vi "LoadConfigPhospho.vi"(8 "configuration file path":path caption="chemin du fichier de configuration") -> (0 "Acquisition properties":T2, 1 "Associated files":T1, 3 "Pulse properties":T3={"N pulses"=0, "Samples"=0, "Last samples"=0, "AO pulse ticks"=0, "Skip samples"=0, "N samples/decay"=0, "Sliding Step \n(nb pulses)"=0, "Slidiing window\n (nb pulses)"=0, "Interpoints \ninterval (ms)"=100.0, "Mean and Time-Lapsed on Point Number"=0, "Number of points"=0, "Repeat \neach point"=8, "Oxygen dye type"=10106, "Interpulse Interval"=0.0, "N samples/ decay min"=0} {"Oxygen dye type" items=["PtP-C343 (30 kDa)", "PtP-C343 (65 KDa)"]; "Repeat \neach point" min=2 step=1})   [LabVIEW 2013, in "Phosphorescence - Mode.lvlib"]
uses:
  Phosphorescence - Mode.lvlib
  <vilib>/Utility/config.llb/Read Key (I32).vi
  <vilib>/Utility/config.llb/Read Key (Double).vi
  <vilib>/Utility/config.llb/Read Key (String).vi
  <vilib>/Utility/config.llb/NI_LVConfig.lvlib
  File management.lvlib
panel:
  out "Wait":i32=30
  in  "TDMS path":string
  out "N samples/ decay min":i32
  out "Interpulse Interval":dbl
  in  "Oxygen dye type":i16(ring)=10106 items=["PtP-C343 (30 kDa)", "PtP-C343 (65 KDa)"]
  in  "Timing file":string
  in  "Results file":string
  in  "Raw Images file":string[][](array[string])
  in  "Repeat \neach point":i32
  in  "Number of points":i32
  in  "Mean and Time-Lapsed on Point Number":i32
  in  "Interpoints \ninterval (ms)":dbl
  in  "Reference text file":string
  in  "Reference image files":string[](array[string])
  in  "Mean and fit file":string
  out "Selection coordinates":dbl[](array[numeric])=[0.5875, 0.6937500000000001, 0.9437500000000001, 0.9750000000000001, 0.5875, 0.7364583333333334, 0.5916666666666667, 0.696875, 0.9333333333333333, 0.6937500000000001, 0.9437500000000001, 0.7208333333333333, 0.7822916666666666, 0.9750000000000001, 0.7562500000000001, 0.971875, 0.5875, 0.7364583333333334]
  out "Pictures coordinates":dbl[](array[numeric])=[0.5875, 0.6937500000000001, 0.9437500000000001, 0.9750000000000001, 0.5875, 0.7364583333333334, 0.5916666666666667, 0.696875, 0.9333333333333333, 0.6937500000000001, 0.9437500000000001, 0.7208333333333333, 0.7822916666666666, 0.9750000000000001, 0.7562500000000001, 0.971875, 0.5875, 0.7364583333333334]
  out "pwr_rel":dbl(slide)=0.01 min=0.01 max=1.0 step=0.005 scale=0.01..1.0 scale format="%.2f"
  out "Channel Acquired":i32 min=0 max=1 step=1
  out "scan rate (kHz)":dbl=1000.0 caption="Rate (kHz)"
  out "Last samples":i32=5
  out "Sliding Step \n(nb pulses)":i32=8 min=2 step=1
  out "Slidiing window\n (nb pulses)":i32=8 min=2 step=1
  out "Skip samples":i32=12
  out "Samples":i32=1500 caption="Total scans"
  out "N samples/decay":i32=150
  out "pulse ticks":i32=8 min=2 step=1
  out "N pulses":i32=10
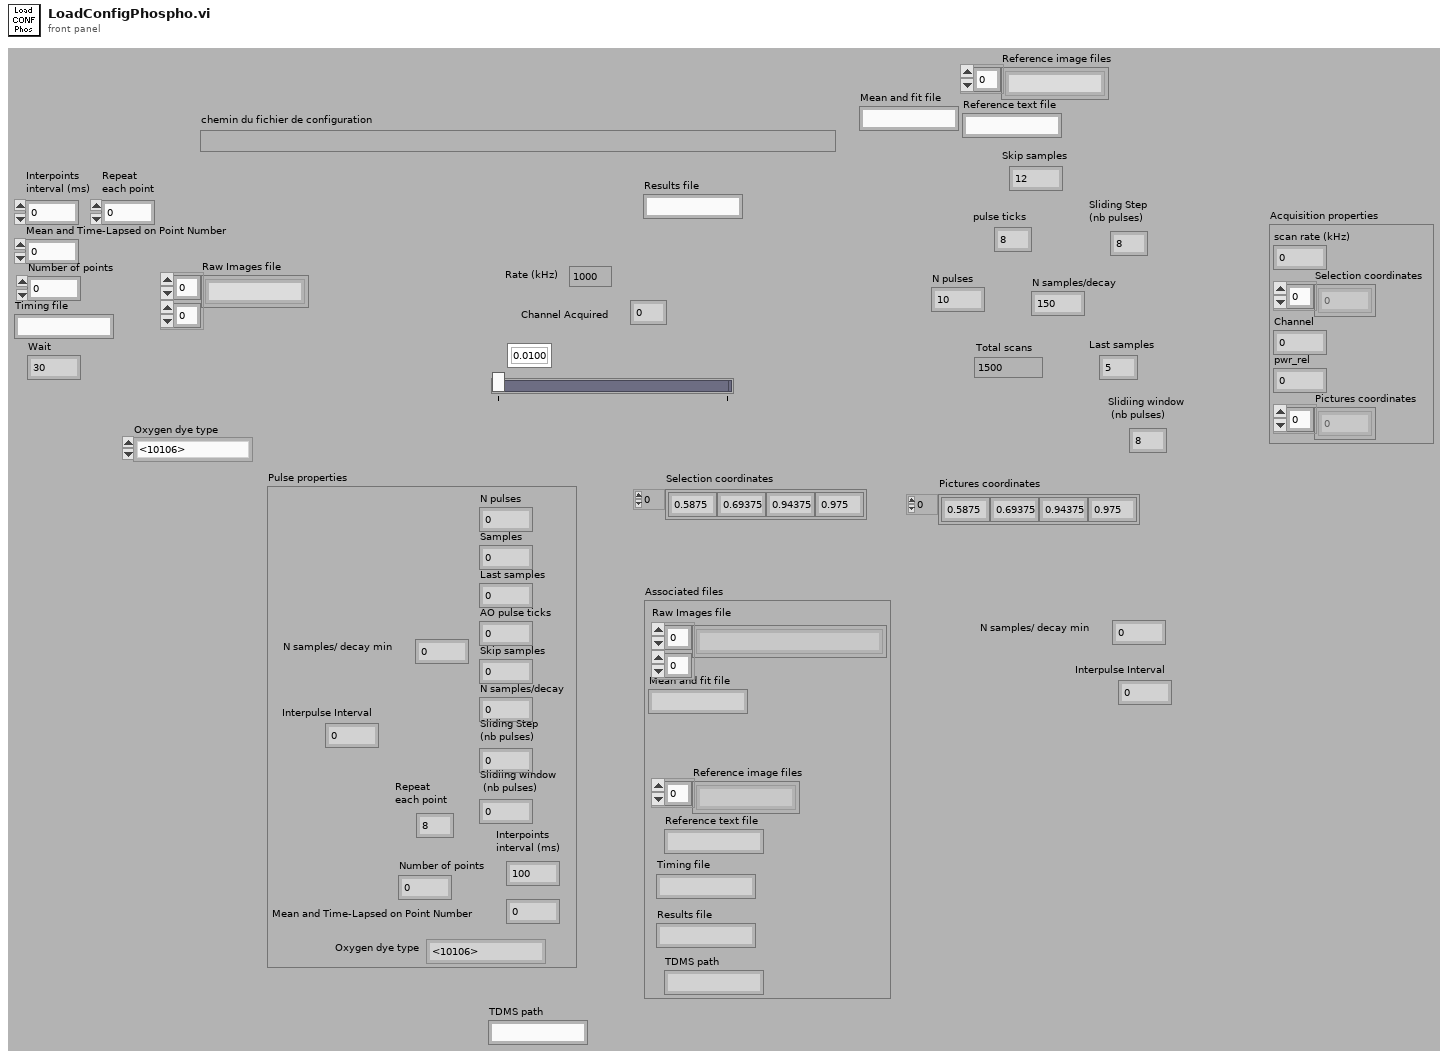
[diagram p1: front panel]
types:
  T1 = cluster{"Mean and fit file":string, "Reference image files":string[], "Reference text file":string, "Results file":string, "Timing file":string, "Raw Images file":string[][], "TDMS path":string}
  T2 = cluster{"scan rate (kHz)":dbl, "Selection coordinates":dbl[], "Channel":i32, "pwr_rel":dbl, "Pictures coordinates":dbl[]}
  T3 = cluster{"N pulses":i32, "Samples":i32, "Last samples":i32, "AO pulse ticks":i32, "Skip samples":i32, "N samples/decay":i32, "Sliding Step \n(nb pulses)":i32, "Slidiing window\n (nb pulses)":i32, "Interpoints \ninterval (ms)":dbl, "Mean and Time-Lapsed on Point Number":i32, "Number of points":i32, "Repeat \neach point":i32, "Oxygen dye type":i16, "Interpulse Interval":dbl, "N samples/ decay min":i32}
  T4 = typedef "NI_LVConfig.lvlib/Config Data RefNum.ctl" = refnum<k1>
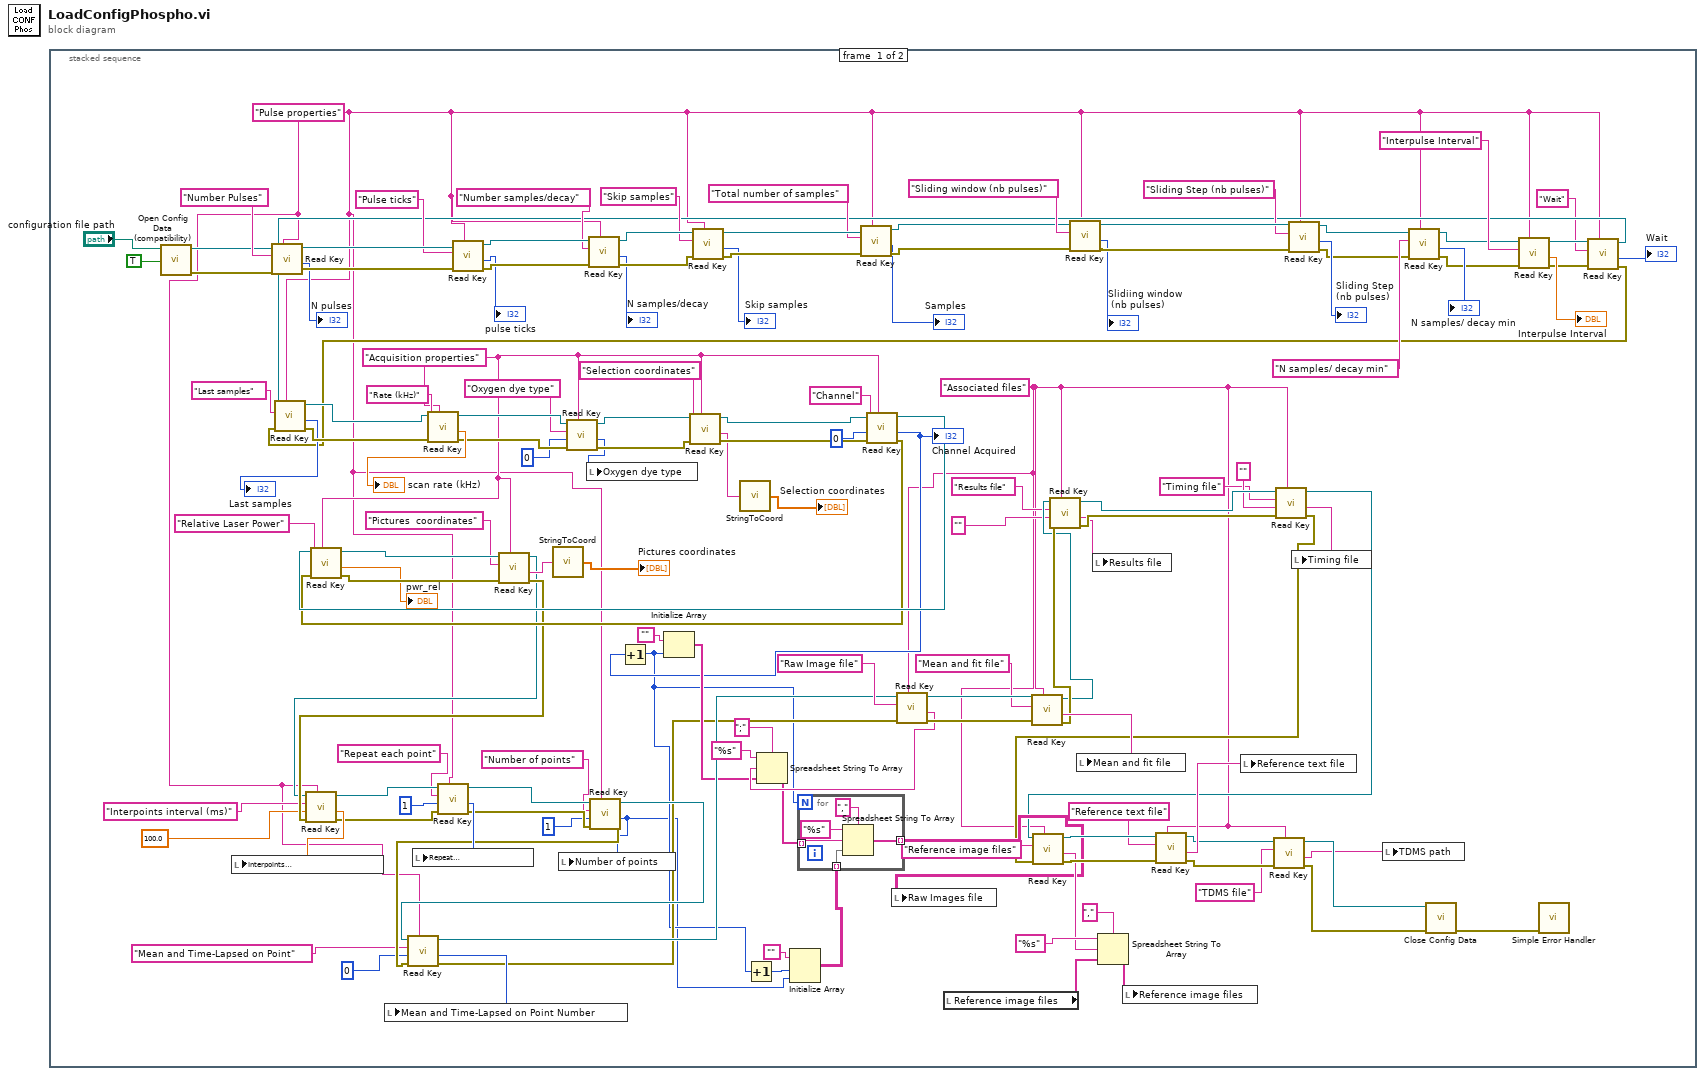
[diagram p0: block diagram]
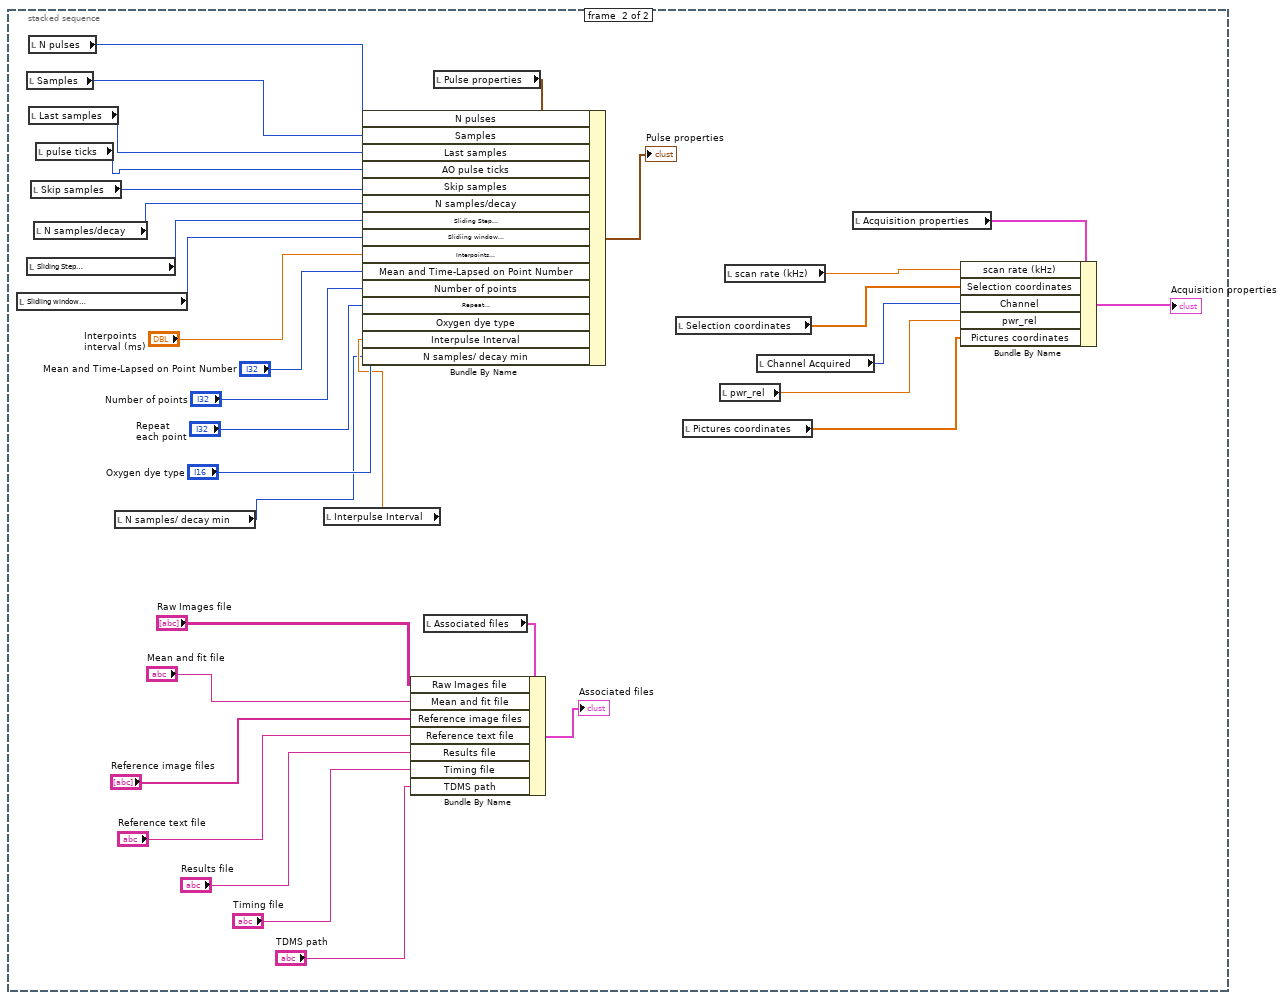
[diagram p2: hidden frame]
diagram:
  n1 = stacked-sequence {
    frame #0 {
      w9 = "Associated files" ("key")
      w29 = "Acquisition properties" ("section")
      w1 = "Pulse properties" ("section")
      n2 = call <vilib>:"Open Config Data (compatibility).vi"("create file if necessary (T)"=TRUE ("create file if necessary? (T)"), "configuration file path"="configuration file path") -> ("error out"=w113:errorcluster, "refnum"=w112:T4)  [unwired: 7 in, 1 out]
      n3 = call-poly <vilib>:"Read Key.vi"("section"=w1, "error in (no error)"=w113, "key"="Number Pulses", "refnum"=w112) -> ("error out"=w124:errorcluster, "value"=→"N pulses":i32, "refnum out"=w119:T4)  [unwired: 1 in, 4 out]
      n4 = call-poly <vilib>:"Read Key.vi"("section"=w1, "error in (no error)"=w124, "key"="Pulse ticks", "refnum"=w119) -> ("error out"=w123:errorcluster, "value"=→"pulse ticks":i32, "refnum out"=w118:T4)  [unwired: 1 in, 4 out]
      n5 = call-poly <vilib>:"Read Key.vi"("section"=w1, "error in (no error)"=w123, "key"="Number samples/decay", "refnum"=w118) -> ("error out"=w122:errorcluster, "value"=→"N samples/decay":i32, "refnum out"=w121:T4)  [unwired: 1 in, 4 out]
      n6 = call-poly <vilib>:"Read Key.vi"("section"=w1, "error in (no error)"=w122, "key"="Skip samples", "refnum"=w121) -> ("error out"=w130:errorcluster, "value"=→"Skip samples":i32, "refnum out"=w129:T4)  [unwired: 1 in, 4 out]
      n7 = call-poly <vilib>:"Read Key.vi"("section"=w1, "error in (no error)"=w130, "key"="Total number of samples", "refnum"=w129) -> ("error out"=w107:errorcluster, "value"=→"Samples":i32, "refnum out"=w108:T4)  [unwired: 1 in, 4 out]
      n8 = local read "Reference image files"() -> (w85:string[])
      n9 = call-poly <vilib>:"Read Key.vi"("section"=w1, "error in (no error)"=w107, "key"="Sliding window (nb pulses)", "refnum"=w108) -> ("error out"=w142:errorcluster, "value"=→"Slidiing window\n (nb pulses)":i32, "refnum out"=w141:T4)  [unwired: 1 in, 4 out]
      n10 = call-poly <vilib>:"Read Key.vi"("section"=w1, "error in (no error)"=w142, "key"="Sliding Step (nb pulses)", "refnum"=w141) -> ("error out"=w18:errorcluster, "value"=→"Sliding Step \n(nb pulses)":i32, "refnum out"=w19:T4)  [unwired: 1 in, 4 out]
      n11 = call-poly <vilib>:"Read Key.vi"("section"=w1, "error in (no error)"=w18, "key"="N samples/ decay min", "refnum"=w19) -> ("error out"=w17:errorcluster, "value"=→"N samples/ decay min":i32, "refnum out"=w20:T4)  [unwired: 1 in, 4 out]
      n12 = call-poly <vilib>:"Read Key.vi"("section"=w1, "error in (no error)"=w17, "key"="Interpulse Interval", "refnum"=w20) -> ("error out"=w5:errorcluster, "value"=→"Interpulse Interval":dbl, "refnum out"=w3:T4)  [unwired: 1 in, 4 out]
      n13 = call-poly <vilib>:"Read Key.vi"("section"=w1, "error in (no error)"=w5, "key"="Wait", "refnum"=w3) -> ("error out"=w6:errorcluster, "value"=→"Wait":i32, "refnum out"=w4:T4)  [unwired: 2 in, 3 out]
      n14 = call-poly <vilib>:"Read Key.vi"("section"=w1, "error in (no error)"=w6, "key"="Last samples", "refnum"=w4) -> ("error out"=w144:errorcluster, "value"=→"Last samples":i32, "refnum out"=w126:T4)  [unwired: 1 in, 4 out]
      n15 = call-poly <vilib>:"Read Key.vi"("section"=w29, "error in (no error)"=w144, "key"="Rate (kHz)", "refnum"=w126) -> ("error out"=w33:errorcluster, "value"=→"scan rate (kHz)":dbl, "refnum out"=w30:T4)  [unwired: 2 in, 3 out]
      n16 = call-poly <vilib>:"Read Key.vi"("section"=w29, "error in (no error)"=w33, "default value"=0, "key"="Oxygen dye type", "refnum"=w30) -> ("error out"=w32:errorcluster, "value"=w27:i32, "refnum out"=w31:T4)  [unwired: 4 out]
      n17 = local write "Oxygen dye type"(w27) -> ()
      n18 = call-poly <vilib>:"Read Key.vi"("section"=w29, "error in (no error)"=w32, "key"="Selection coordinates", "refnum"=w31) -> ("error out"=w133:errorcluster, "value"=w15:string, "refnum out"=w132:T4)  [unwired: 2 in, 3 out]
      n19 = call "StringToCoord.vi"("String coordinates"=w15) -> ("coordinates"=→"Selection coordinates":dbl[])
      n20 = call-poly <vilib>:"Read Key.vi"("section"=w29, "error in (no error)"=w133, "default value"=0, "key"="Channel", "refnum"=w132) -> ("error out"=w135:errorcluster, "value"=w39:i32, "refnum out"=w136:T4)  [unwired: 4 out]
      "Channel Acquired" <- w39
      n21 = call-poly <vilib>:"Read Key.vi"("section"=w29, "error in (no error)"=w135, "key"="Relative Laser Power", "refnum"=w136) -> ("error out"=w139:errorcluster, "value"=→"pwr_rel":dbl, "refnum out"=w138:T4)  [unwired: 1 in, 4 out]
      n22 = call-poly <vilib>:"Read Key.vi"("section"=w29, "error in (no error)"=w139, "key"="Pictures  coordinates", "refnum"=w138) -> ("error out"=w73:errorcluster, "value"=w79:string, "refnum out"=w72:T4)  [unwired: 2 in, 3 out]
      n23 = call-poly <vilib>:"Read Key.vi"("section"=w1, "error in (no error)"=w73, "default value"=100.0, "key"="Interpoints interval (ms)", "refnum"=w72) -> ("error out"=w74:errorcluster, "value"=w78:dbl, "refnum out"=w71:T4)  [unwired: 4 out]
      n24 = local write "Interpoints \ninterval (ms)"(w78) -> ()
      n25 = call-poly <vilib>:"Read Key.vi"("section"=w1, "error in (no error)"=w74, "default value"=1, "key"="Repeat each point", "refnum"=w71) -> ("error out"=w75:errorcluster, "value"=w77:i32, "refnum out"=w70:T4)  [unwired: 4 out]
      n26 = local write "Repeat \neach point"(w77) -> ()
      n27 = call "StringToCoord.vi"("String coordinates"=w79) -> ("coordinates"=→"Pictures coordinates":dbl[])
      n28 = call-poly <vilib>:"Read Key.vi"("section"=w1, "error in (no error)"=w75, "default value"=1, "key"="Number of points", "refnum"=w70) -> ("error out"=w76:errorcluster, "value"=w35:i32, "refnum out"=w69:T4)  [unwired: 4 out]
      n29 = call-poly <vilib>:"Read Key.vi"("section"=w1, "error in (no error)"=w76, "default value"=0, "key"="Mean and Time-Lapsed on Point", "refnum"=w69) -> ("error out"=w42:errorcluster, "value"=w67:i32, "refnum out"=w68:T4)  [unwired: 4 out]
      n30 = local write "Mean and Time-Lapsed on Point Number"(w67) -> ()
      n31 = local write "Number of points"(w35) -> ()
      n32 = Increment(x=w39) -> (x+1=w36:i32)
      n33 = Initialize Array("", w36) -> (w44:string[])
      n34 = Increment(x=w36) -> (x+1=w38:i32)
      n35 = Initialize Array("", w38, w35) -> (w34:string[][])
      n36 = call-poly <vilib>:"Read Key.vi"("section"=w9, "error in (no error)"=w42, "key"="Raw Image file", "refnum"=w68) -> ("error out"=w104:errorcluster, "value"=w46:string, "refnum out"=w106:T4)  [unwired: 2 in, 3 out]
      n37 = Spreadsheet String To Array(delimiter (Tab)=";" ("séparateur (Tabulation)"), format string="%s" ("chaîne de format"), spreadsheet string=w46, array type (2D Dbl)=w44) -> (array=w41:string[])
      n38 = for {
        N: w36 -> [_]
        tunnel: w41 -> [w147] mode=indexing
        tunnel: [w146] -> w40 mode=indexing
        tunnel: w34 -> [w145] mode=indexing
        n39 = Spreadsheet String To Array(delimiter (Tab)="," ("séparateur (Tabulation)"), format string="%s" ("chaîne de format"), spreadsheet string=w147, array type (2D Dbl)=w145) -> (array=w146:string[])
      }
      n40 = local write "Raw Images file"(w40) -> ()
      n41 = call-poly <vilib>:"Read Key.vi"("section"=w9, "error in (no error)"=w104, "key"="Mean and fit file", "refnum"=w106) -> ("error out"=w56:errorcluster, "value"=w97:string, "refnum out"=w55:T4)  [unwired: 2 in, 3 out]
      n42 = call-poly <vilib>:"Read Key.vi"("section"=w9, "error in (no error)"=w56, "default value"="", "key"="Results file", "refnum"=w55) -> ("error out"=w57:errorcluster, "value"=w54:string, "refnum out"=w58:T4)  [unwired: 1 in, 3 out]
      n43 = local write "Mean and fit file"(w97) -> ()
      n44 = local write "Results file"(w54) -> ()
      n45 = call-poly <vilib>:"Read Key.vi"("section"=w9, "error in (no error)"=w57, "default value"="", "key"="Timing file", "refnum"=w58) -> ("error out"=w24:errorcluster, "value"=w53:string, "refnum out"=w25:T4)  [unwired: 1 in, 3 out]
      n46 = call-poly <vilib>:"Read Key.vi"("section"=w9, "error in (no error)"=w24, "key"="Reference image files", "refnum"=w25) -> ("error out"=w103:errorcluster, "value"=w82:string, "refnum out"=w105:T4)  [unwired: 2 in, 3 out]
      n47 = Spreadsheet String To Array(delimiter (Tab)="," ("séparateur (Tabulation)"), format string="%s" ("chaîne de format"), spreadsheet string=w82, array type (2D Dbl)=w85) -> (array=w86:string[])
      n48 = local write "Reference image files"(w86) -> ()
      n49 = call-poly <vilib>:"Read Key.vi"("section"=w9, "error in (no error)"=w103, "key"="Reference text file", "refnum"=w105) -> ("error out"=w14:errorcluster, "value"=w98:string, "refnum out"=w13:T4)  [unwired: 2 in, 3 out]
      n50 = local write "Reference text file"(w98) -> ()
      n51 = call-poly <vilib>:"Read Key.vi"("section"=w9, "error in (no error)"=w14, "key"="TDMS file", "refnum"=w13) -> ("error out"=w12:errorcluster, "value"=w10:string, "refnum out"=w11:T4)  [unwired: 2 in, 3 out]
      n52 = local write "Timing file"(w53) -> ()
      n53 = local write "TDMS path"(w10) -> ()
      n54 = call <vilib>:"Close Config Data.vi"("error in (no error)"=w12, "refnum"=w11) -> ("error out"=w143:errorcluster)  [unwired: 1 in, 8 out]
      n55 = call <vilib>:"Simple Error Handler.vi"("error in (no error)"=w143) -> ()  [unwired: 1 in, 8 out]
    }
    frame #1 {
      n56 = local read "Slidiing window\n (nb pulses)"() -> (w173:i32)
      n57 = local read "Samples"() -> (w179:i32)
      n58 = local read "Sliding Step \n(nb pulses)"() -> (w174:i32)
      n59 = local read "N pulses"() -> (w180:i32)
      n60 = local read "Last samples"() -> (w178:i32)
      n61 = local read "Skip samples"() -> (w176:i32)
      n62 = local read "N samples/decay"() -> (w175:i32)
      n63 = local read "pulse ticks"() -> (w177:i32)
      n64 = local read "N samples/ decay min"() -> (w151:i32)
      n65 = local read "Interpulse Interval"() -> (w152:dbl)
      n66 = local read "Associated files"() -> (w172:T1)
      n67 = Bundle By Name(cluster=w172, "Raw Images file"="Raw Images file", "Mean and fit file"="Mean and fit file", "Reference image files"="Reference image files", "Reference text file"="Reference text file", "Results file"="Results file", "Timing file"="Timing file", "TDMS path"="TDMS path") -> (→"Associated files":T1)
      n68 = local read "Pulse properties"() -> (w182:T3)
      n69 = Bundle By Name(cluster=w182, "N pulses"=w180, "Samples"=w179, "Last samples"=w178, "AO pulse ticks"=w177, "Skip samples"=w176, "N samples/decay"=w175, "Sliding Step \n(nb pulses)"=w174, "Slidiing window\n (nb pulses)"=w173, "Interpoints \ninterval (ms)"="Interpoints \ninterval (ms)", "Mean and Time-Lapsed on Point Number"="Mean and Time-Lapsed on Point Number", "Number of points"="Number of points", "Repeat \neach point"="Repeat \neach point", "Oxygen dye type"="Oxygen dye type", "Interpulse Interval"=w152, "N samples/ decay min"=w151) -> (→"Pulse properties":T3)
      n70 = local read "Selection coordinates"() -> (w164:dbl[])
      n71 = local read "Pictures coordinates"() -> (w161:dbl[])
      n72 = local read "pwr_rel"() -> (w162:dbl)
      n73 = local read "scan rate (kHz)"() -> (w165:dbl)
      n74 = local read "Channel Acquired"() -> (w163:i32)
      n75 = local read "Acquisition properties"() -> (w167:T2)
      n76 = Bundle By Name(cluster=w167, "scan rate (kHz)"=w165, "Selection coordinates"=w164, "Channel"=w163, "pwr_rel"=w162, "Pictures coordinates"=w161) -> (→"Acquisition properties":T2)
    }
  }
